vi "text_message_to_ollama_message.vi"(1 "message":T1) -> (0 "messages out":cluster{"role":string, "content":string}[](array[cluster]))   [LabVIEW 2020, in "llm_ollama_chatmodels.lvclass"]
uses:
  llm_ollama_chatmodels.lvclass
  message_text/message.ctl
  message_text/message_text.lvclass
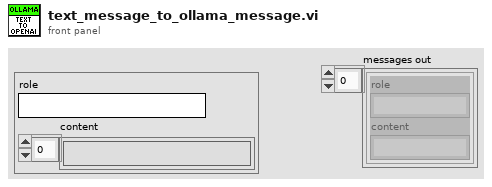
[diagram p1: front panel]
types:
  T1 = typedef "message_text.lvclass/message.ctl" = cluster{"role":string, "content":string[]}
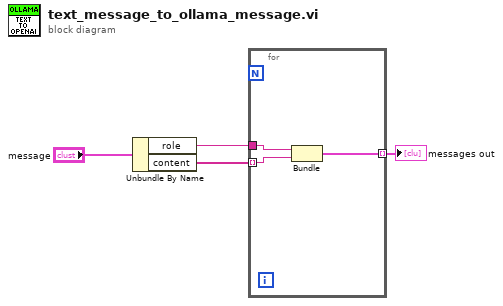
[diagram p0: block diagram]
diagram:
  n1 = Unbundle By Name("message") -> ("role"=w3:string, "content"=w2:string[])
  n2 = for {
    tunnel: w3 -> [w7]
    tunnel: w2 -> [w6] mode=indexing
    tunnel: [w5] -> w1 mode=indexing
    n3 = Bundle("role"=w7, "text"=w6) -> (w5:cluster{"role":string, "text":string})  [unwired: 1 in]
  }
  "messages out" <- w1
